vi "Conti_SendReceive.vi"(6 "error source":string="Diagnostic Service.vi", 8 "error in (no error)":errorcluster, 9 "data in":u8[](array[numeric]), 10 "require response?":bool=TRUE, 11 "diag ref in":T1) -> (0 "error out":errorcluster, 1 "data out":u8[](array[numeric]), 2 "error code":u8, 3 "diag ref out":T1)   [LabVIEW 2015, in "Diagnostics Addon Engine.lvlib"]
uses:
  <vilib>/Automotive Diagnostic Command Set/Diagnostic Transport.llb/Diag Reference.ctl
  <vilib>/Automotive Diagnostic Command Set/Diagnostic Transport.llb/Transport Protocol Selector.ctl
  <vilib>/Automotive Diagnostic Command Set/Diagnostic Transport.llb/Diag CAN Frame Log.ctl
  <vilib>/Automotive Diagnostic Command Set/Diagnostic Transport.llb/Diag Globals.vi
  Diagnostics Addon Engine.lvlib
  <vilib>/addons/Automotive Diagnostic Command Set/NI_Automotive Diagnostic Command Set.lvlib
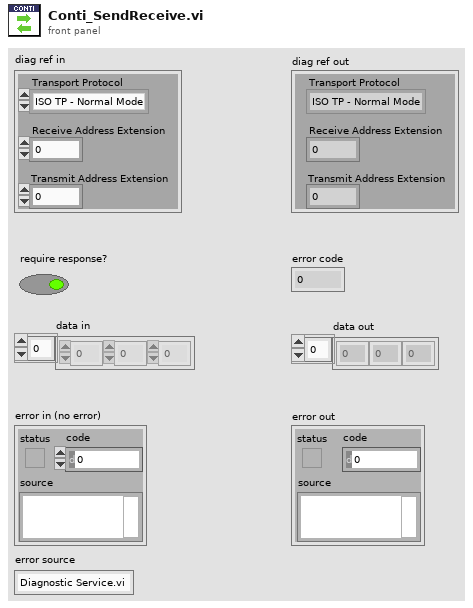
[diagram p1: front panel]
types:
  T1 = typedef "NI_Automotive Diagnostic Command Set.lvlib/Diag Reference.ctl" = cluster{"Diag CAN Handle":u32, "Transport Protocol":T2, "Receive Address Extension":u8, "Transmit Address Extension":u8, "Receive CAN Id":u32, "Transmit CAN Id":u32, "Diag CAN Queue":refnum<queue>, "Log Frames ?":bool, "My TP Address":u8, "Other TP Address":u8, "T1":u16, "T2":u16, "T3":u16, "T4":u16, "Tx SN":u8, "Block Size":u8, "Rx SN":u8, "VW TP Initialized?":bool, "Tx block no":u8, "baud rate":u32, "Interface":string, "Channel Diag CAN Handle":u32, "UDP Connection ID":refnum<k16>, "TCP Connection ID":refnum<k5>, "Target IP Addr":u32, "Source Address":u16, "Target Address":u16, "Send Header NACK?":bool, "DLL Handle":u32, "NAD":u8, "Time Stamp read first":dbl, "Time Stamp read last":dbl, "Time Stamp write first":dbl, "Time Stamp write last":dbl, "Time Stamp write":dbl, "Time Stamp read":dbl}
  T2 = typedef "NI_Automotive Diagnostic Command Set.lvlib/Transport Protocol Selector.ctl" = enum16{"ISO TP - Normal Mode", "ISO TP - Mixed Mode", "VW TP 2.0", "Diagnostics on IP", "ISO TP LIN"}
  T3 = typedef "NI_Automotive Diagnostic Command Set.lvlib/Diag Globals.ctl" = cluster{"Timeout FC (Bs)":u32, "Timeout CF (Cr)":u32, "Timeout Diag Command":u32, "Receive Block Size (BS)":u8, "Wait Time CF (STmin)":u8, "Max Waits (N_WFTmax)":u8, "Waits to Send (N_WAIT)":i32, "Time between Waits (TW)":u32, "Fill CAN Frames?":bool, "Fill Byte":u32, "Invalid Response as Error?":bool, "Max RspPending Count":u32, "VWTP Command Timeout":u32, "Transport Protocol":T2, "Diag CAN Handle":u32, "DLL Handle":u32}
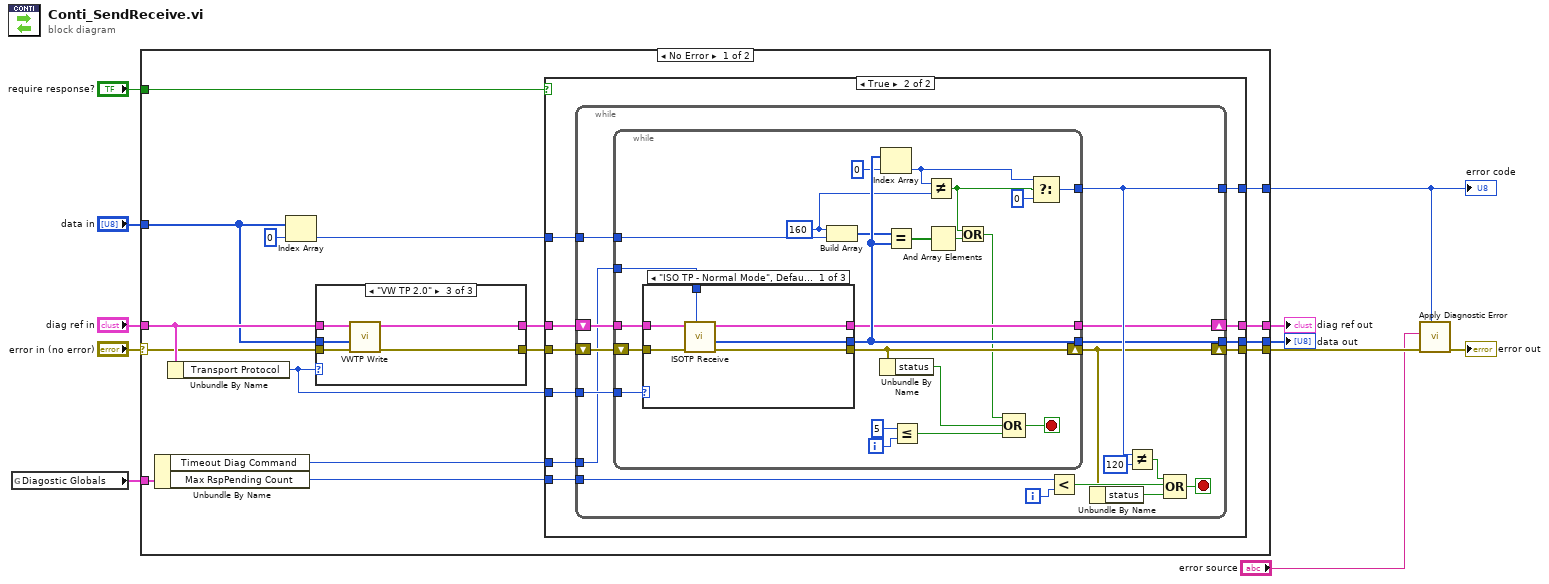
[diagram p0: block diagram]
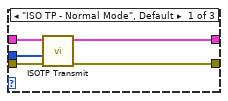
[diagram p2: hidden frame]
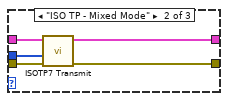
[diagram p3: hidden frame]
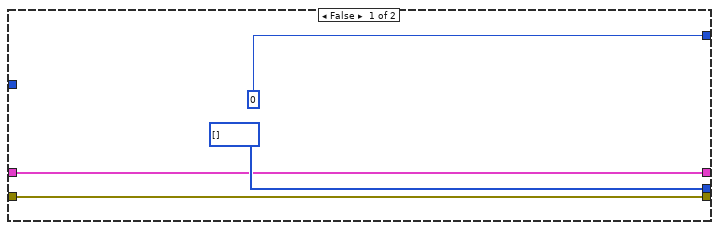
[diagram p4: hidden frame]
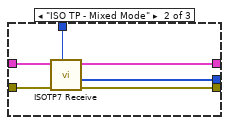
[diagram p5: hidden frame]
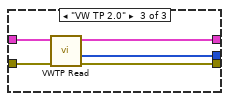
[diagram p6: hidden frame]
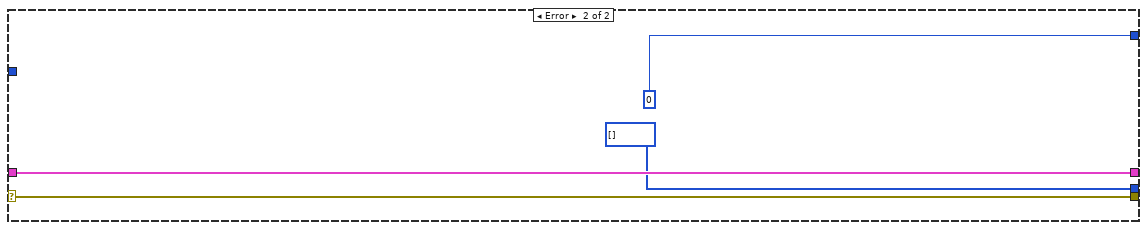
[diagram p7: hidden frame]
diagram:
  n1 = global read "Diag Globals.vi" "Diagostic Globals"() -> (w2:T3)
  n2 = case shown="No Error" "error in (no error)" {
    selector: "error in (no error)" -> [w20 w115]
    tunnel: "data in" -> [w19 _]
    tunnel: [w27 u8[] [] ("data out")] -> w5
    tunnel: [w26 w116] -> w1
    tunnel: [w25 w115] -> w11
    tunnel: "diag ref in" -> [w21 w116]
    tunnel: [w24 u8 0 ("error code")] -> w8
    tunnel: "require response?" -> [w23 _]
    tunnel: w2 -> [w16 _]
    frame No Error {
      n3 = Unbundle By Name(w16) -> ("Timeout Diag Command"=w12:u32, "Max RspPending Count"=w15:u32)
      n4 = Unbundle By Name(w21) -> ("Transport Protocol"=w13:T2)
      n5 = Index Array(array=w19, index=0) -> (element=w14:u8)
      n6 = case shown="\"VW TP 2.0\"" w13 {
        tunnel: w20 -> [w32 w37 w41]
        tunnel: w19 -> [w31 w36 w38]
        tunnel: [w29 w34 w40] -> w17
        tunnel: w21 -> [w30 w35 w42]
        tunnel: [w28 w33 w39] -> w18
        frame "ISO TP - Normal Mode", Default {
          n7 = call <vilib>:"ISOTP Transmit.vi"("error in (no error)"=w32, "data"=w31, "diag ref in"=w30) -> ("error out"=w28:errorcluster, "diag ref out"=w29:T1)  [unwired: 7 in]
        }
        frame "ISO TP - Mixed Mode" {
          n8 = call <vilib>:"ISOTP7 Transmit.vi"("error in (no error)"=w37, "data"=w36, "diag ref in"=w35) -> ("error out"=w33:errorcluster, "diag ref out"=w34:T1)  [unwired: 7 in]
        }
        frame "VW TP 2.0" {
          n9 = call <vilib>:"VWTP Write.vi"("error in"=w41, "data in"=w38, "diag ref in"=w42) -> ("error out"=w39:errorcluster, "diag ref out"=w40:T1)  [unwired: 7 in]
        }
      }
      n10 = case shown="True" w23 {
        tunnel: [u8[] [] ("data out") w56] -> w27
        tunnel: [w45 w55] -> w26
        tunnel: [w44 w54] -> w25
        tunnel: w17 -> [w45 w53]
        tunnel: w18 -> [w44 w52]
        tunnel: [u8 0 ("error code") w51] -> w24
        tunnel: w15 -> [_ w50]
        tunnel: w14 -> [_ w49]
        tunnel: w13 -> [_ w48]
        tunnel: w12 -> [_ w47]
        frame False {
        }
        frame True {
          n11 = while {
            tunnel: [w61] -> w56
            shift-right: [w60] -> w54
            shift-left: w52 -> [w65]
            tunnel: [w62] -> w51
            shift-right: [w59] -> w55
            shift-left: w53 -> [w64]
            tunnel: w50 -> [w66]
            tunnel: w49 -> [w63]
            tunnel: w48 -> [w58]
            tunnel: w47 -> [w57]
            i -> [w68]
            stop <- w71 stop-if-true
            n12 = while {
              tunnel: [w88] -> w61
              tunnel: [w85] -> w59
              tunnel: w64 -> [w89]
              tunnel: w63 -> [w91]
              tunnel: [w87] -> w62
              shift-right: [w86] -> w60
              shift-left: w65 -> [w90]
              tunnel: w58 -> [w82]
              tunnel: w57 -> [w81]
              i -> [w92]
              stop <- w95 stop-if-true
              w79 = u8 160 ("element")
              n13 = case shown="\"ISO TP - Normal Mode\", Default" w82 {
                tunnel: w90 -> [w96 w102 w111]
                tunnel: [w101 w107 w108] -> w88
                tunnel: [w100 w106 w109] -> w85
                tunnel: w89 -> [w97 w103 w112]
                tunnel: [w99 w105 w110] -> w86
                tunnel: w81 -> [w98 w104 _]
                frame "ISO TP - Normal Mode", Default {
                  n14 = call <vilib>:"ISOTP Receive.vi"("timeout [ms]"=w98, "error in (no error)"=w96, "diag ref in"=w97) -> ("error out"=w99:errorcluster, "data"=w101:u8[], "diag ref out"=w100:T1)  [unwired: 6 in]
                }
                frame "ISO TP - Mixed Mode" {
                  n15 = call <vilib>:"ISOTP7 Receive.vi"("timeout [ms]"=w104, "error in (no error)"=w102, "diag ref in"=w103) -> ("error out"=w105:errorcluster, "data"=w107:u8[], "diag ref out"=w106:T1)  [unwired: 6 in]
                }
                frame "VW TP 2.0" {
                  n16 = call <vilib>:"VWTP Read.vi"("error in"=w111, "diag ref in"=w112) -> ("error out"=w110:errorcluster, "data out"=w108:u8[], "diag ref out"=w109:T1)  [unwired: 7 in]
                }
              }
              n17 = Build Array(w79, w91) -> (w80:u8[])
              n18 = Unbundle By Name(w86) -> ("status"=w83:bool)
              n19 = Index Array(array=w88, index=0) -> (element=w74:u8)
              n20 = Equal?(x=w80, y=w88) -> (x = y?=w77:bool[])
              n21 = Less Or Equal?(x=5, y=w92) -> (x <= y?=w93:bool)
              n22 = Not Equal?(x=w74, y=w79) -> (x != y?=w75:bool)
              n23 = And Array Elements(Boolean array=w77) -> (logical AND=w76:bool)
              n24 = Or(x=w75, y=w76) -> (x .or. y?=w84:bool)
              n25 = Compound Arithmetic op=OR(w84, w83, w93) -> (w95:bool)
              n26 = Select(t=w74, s=w75, f=u8 0) -> (s? t:f=w87:u8)
            }
            n27 = Less?(x=w66, y=w68) -> (x < y?=w67:bool)
            n28 = Unbundle By Name(w60) -> ("status"=w70:bool)
            n29 = Not Equal?(x=w62, y=u8 120) -> (x != y?=w69:bool)
            n30 = Compound Arithmetic op=OR(w69, w67, w70) -> (w71:bool)
          }
        }
      }
    }
    frame Error {
    }
  }
  "data out" <- w5
  "error code" <- w8
  "diag ref out" <- w1
  n31 = call <vilib>:"Apply Diagnostic Error.vi"("error code"=w8, "error in (no error)"=w11, "error source"="error source") -> ("error out"=→"error out":errorcluster)  [unwired: 8 in]
